vi "Remove Ignored Internals.vi"(11 "Internals in":string[](array[string])) -> (3 "Internals out":string[](array[string]))   [LabVIEW 2019, in "Project.Dependencies Finder.lvlib"]
uses:
  Project.Dependencies Finder.lvlib
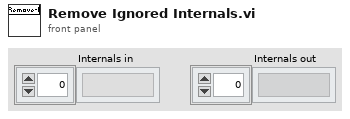
[diagram p1: front panel]
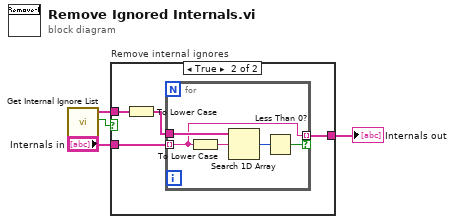
[diagram p0: block diagram]
diagram:
  n1 = call "Get Internal Ignore List.vi"() -> ("Success?"=w1:bool, "Lower case internal ignores"=w4:string[])  [unwired: 10 in]
  n2 = case "Remove internal ignores" shown="True" w1 {
    tunnel: [w5 w7] -> w3
    tunnel: "Internals in" -> [w5 w9]
    tunnel: w4 -> [_ w8]
    frame False {
    }
    frame True {
      n3 = To Lower Case(string=w8) -> (all lower case string=w6:string[])
      n4 = for {
        tunnel: w9 -> [w13] mode=indexing
        tunnel: w6 -> [w14]
        tunnel: [w13] -> w7 mode=indexing if=w11
        n5 = To Lower Case(string=w13) -> (all lower case string=w10:string)
        n6 = Search 1D Array(1D array=w14, element=w10) -> (index of element=w12:i32)  [unwired: 1 in]
        n7 = Less Than 0?(x=w12) -> (x < 0?=w11:bool)
      }
    }
  }
  "Internals out" <- w3
